vi "Server_Response_speed.vi"() -> ()   [LabVIEW 2010]
panel:
  out "?":cluster{dbl[], dbl[]}(graph)
  in  "stop":bool
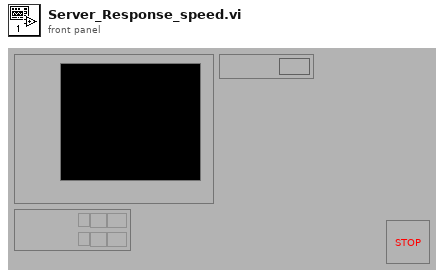
[diagram p1: front panel]
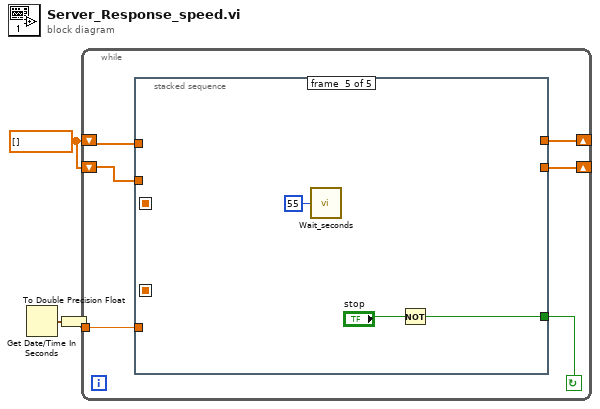
[diagram p0: block diagram]
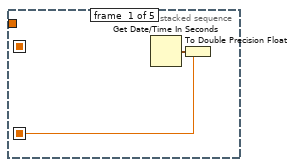
[diagram p2: hidden frame]
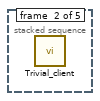
[diagram p3: hidden frame]
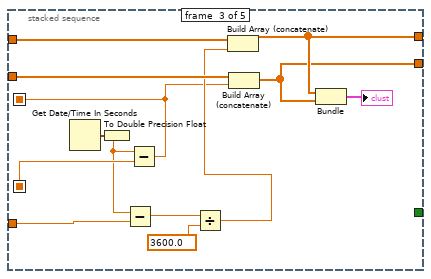
[diagram p4: hidden frame]
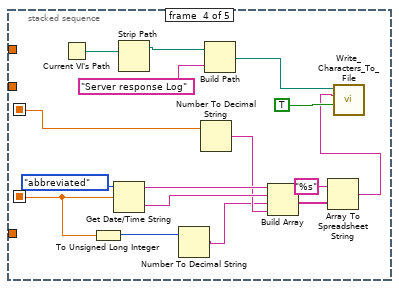
[diagram p5: hidden frame]
diagram:
  w3 = dbl[] []
  n1 = Get Date/Time In Seconds() -> (seconds since 1Jan1904=w1:timestamp)
  n2 = To Double Precision Float(number=w1) -> (double precision float=w2:dbl)
  n3 = while {
    tunnel: w2 -> [w4]
    shift-left: w3 -> [w6]
    shift-right: [w5] -> _
    shift-left: w3 -> [w8]
    shift-right: [w7] -> _
    stop <- w9 continue-if-true
    n4 = stacked-sequence {
      seq-local: [w11 _ _ _ _] -> [_ _ w24 w28 _]
      seq-local: [_ _ w13 _ _] -> [_ _ _ w34 _]
      tunnel: [_ _ _ _ w42] -> w9
      tunnel: w8 -> [_ _ w23 _ _]
      tunnel: [_ _ w21 _ _] -> w7
      tunnel: w6 -> [_ _ w22 _ _]
      tunnel: [_ _ w20 _ _] -> w5
      tunnel: w4 -> [_ _ w17 _ _]
      frame #0 {
        n5 = Get Date/Time In Seconds() -> (seconds since 1Jan1904=w10:timestamp)
        n6 = To Double Precision Float(number=w10) -> (double precision float=w11:dbl)
      }
      frame #1 {
        n7 = call "Trivial_client.vi"() -> ()  [unwired: 4 out]
      }
      frame #2 {
        n8 = Get Date/Time In Seconds() -> (seconds since 1Jan1904=w12:timestamp)
        n9 = To Double Precision Float(number=w12) -> (double precision float=w18:dbl)
        n10 = Subtract(x=w18, y=w17) -> (x-y=w16:dbl)
        n11 = Subtract(x=w18, y=w24) -> (x-y=w13:dbl)
        n12 = Divide(x=w16, y=3600.0) -> (x/y=w14:dbl)
        n13 = Build Array (concatenate)(w23, w14) -> (w21:dbl[])
        n14 = Build Array (concatenate)(w22, w13) -> (w20:dbl[])
        n15 = Bundle(w21, w20) -> (→"?":cluster{dbl[], dbl[]})  [unwired: 1 out]
      }
      frame #3 {
        n16 = Current VI's Path() -> (path=w40:path)
        n17 = To Unsigned Long Integer(number=w28) -> (unsigned 32bit integer=w25:u32)
        n18 = Get Date/Time String(date format (0)=enum16{"short", "long", "abbreviated"}."abbreviated", seconds (now)=w28) -> (date string=w36:string, time string=w35:string)  [unwired: 1 out]
        n19 = Strip Path(path=w40) -> (stripped path=w39:path)  [unwired: 1 out]
        n20 = Number To Decimal String(number=w25) -> (decimal integer string=w26:string)  [unwired: 1 out]
        n21 = Number To Decimal String(number=w34) -> (decimal integer string=w27:string)  [unwired: 1 out]
        n22 = Build Path(base path=w39, name or relative path="Server response Log") -> (appended path=w33:path)
        n23 = Build Array(w36, w35, w26, w27) -> (w31:string[])
        n24 = Array To Spreadsheet String(array=w31, 3:"%s" ("format string")) -> (spreadsheet string=w29:string)  [unwired: 1 out]
        n25 = call "Write_Characters_To_File.vi"("file path (dialog if empty)"=w33, "character string"=w29, "append to file? (new file:F)"=TRUE) -> ()  [unwired: 2 in, 4 out]
      }
      frame #4 {
        n26 = call "Wait_seconds.vi"("Seconds to wait"=u32 55) -> ()
        n27 = Not(x="stop") -> (.not. x?=w42:bool)
      }
    }
  }
